vi "Goo01.vi"() -> ()   [LabVIEW 2014]
uses:
  <vilib>/myRIO/Instrument Drivers/Onboard IO/AI/vis/Read.vi
  <vilib>/myRIO/Instrument Drivers/Onboard IO/AI/vis/Smart Open.vi
  <vilib>/Utility/error.llb/Error Cluster From Error Code.vi
  <vilib>/myRIO/Common/Instrument Driver Framework/myRIO v1.0/AI/vis/myRIO v1.0 Read AI.vi
panel:
  out "웨이브폼 차트":cluster{"Col01 (B/AI1 (Pin 5))":dbl, dbl}(graph)
  out "숫자형":dbl=2.943114933
  out "Col02 (B/AI2 (Pin 7))":dbl=2.980956726
  out "원소의 인덱스":i32
  out "숫자형 2":dbl=2.46582006
  out "Col02 (B/AI2 (Pin 7)) 2":dbl=2.708739957
  # "오른쪽 수평 맞추기"
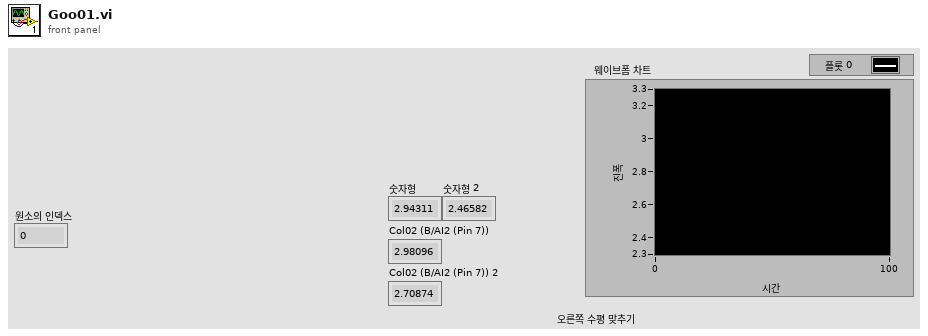
[diagram p1: front panel]
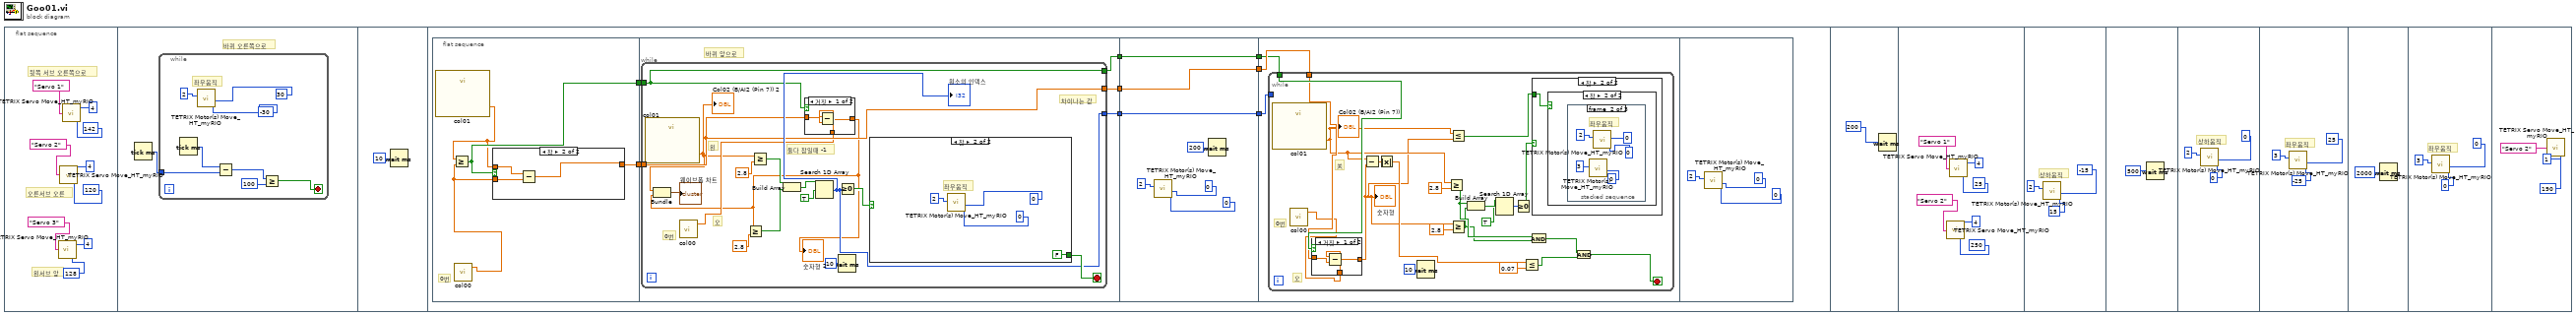
[diagram p0: block diagram]
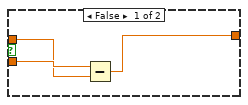
[diagram p2: hidden frame]
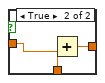
[diagram p3: hidden frame]
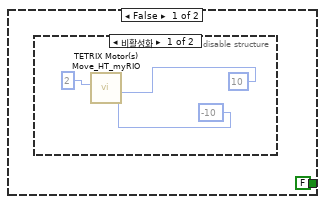
[diagram p4: hidden frame]
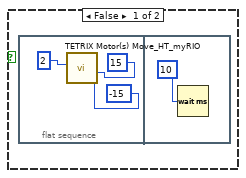
[diagram p6: hidden frame]
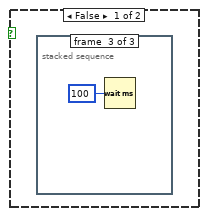
[diagram p7: hidden frame]
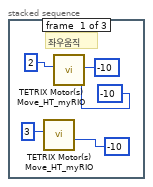
[diagram p8: hidden frame]
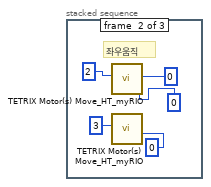
[diagram p9: hidden frame]
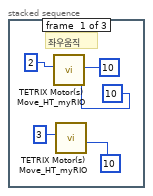
[diagram p10: hidden frame]
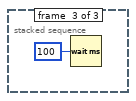
[diagram p11: hidden frame]
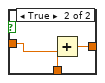
[diagram p12: hidden frame]
diagram:
  n1 = flat-sequence {
    frame #0 {
      # "왼서브 앞"
      # "오른서브 오른"
      # "뒷쪽 서브 오른쪽으로"
      n2 = call <vilib>:"TETRIX Servo Move_HT_myRIO.vi"("Servo Position (0 - 255)"=u8 128, "Controller Daisy Chain Position (1 - 4)"=u8 4, "Select Servo"="Servo 3") -> ()  [unwired: 2 in, 1 out]
      n3 = call <vilib>:"TETRIX Servo Move_HT_myRIO.vi"("Servo Position (0 - 255)"=u8 120, "Controller Daisy Chain Position (1 - 4)"=u8 4, "Select Servo"="Servo 2") -> ()  [unwired: 2 in, 1 out]
      n4 = call <vilib>:"TETRIX Servo Move_HT_myRIO.vi"("Servo Position (0 - 255)"=u8 142, "Controller Daisy Chain Position (1 - 4)"=u8 4, "Select Servo"="Servo 1") -> ()  [unwired: 2 in, 1 out]
    }
    frame #1 {
      # "바퀴 오른쪽으로"
      n5 = Tick Count (ms)() -> (millisecond timer value=w10:u32)
      n6 = while {
        tunnel: w10 -> [w14]
        stop <- w11 stop-if-true
        # "좌우움직"
        n7 = Tick Count (ms)() -> (millisecond timer value=w15:u32)
        n8 = call <vilib>:"TETRIX Motor(s) Move_HT_myRIO.vi"("Motor 2 Power (-100 to 100)\n0 = Stop/Brake\n-128 = Stop/Coast"=i8 -30 ("Motor 2 Power (-100 to 100)\n0 = Stop/Brake\n-128 = Stop/Coast"), "Motor 1 Power (-100 to 100)\n0 = Stop/Brake\n-128 = Stop/Coast"=i8 30 ("Motor 1 Power (-100 to 100)\n0 = Stop/Brake\n-128 = Stop/Coast"), "Controller Daisy Chain Position: 1 - 4"=u8 2) -> ()  [unwired: 6 in, 1 out]
        n9 = Subtract(x=w15, y=w14) -> (x-y=w13:u32)
        n10 = Greater Or Equal?(x=w13, y=u32 100) -> (x >= y?=w11:bool)
      }
    }
    frame #2 {
      n11 = Wait (ms)(milliseconds to wait=u32 10 ("대기 시간(ms)")) -> ()  [unwired: 1 out]
    }
    frame #3 {
      n12 = flat-sequence {
        tunnel: [w31] -> w27
        tunnel: [w30] -> w26
        tunnel: [w42] -> w25
        tunnel: [w41] -> w24
        tunnel: [w40] -> w23
        tunnel: w27 -> [w39]
        tunnel: w26 -> [w38]
        tunnel: w25 -> [w75]
        tunnel: w24 -> [w73]
        tunnel: w23 -> [w74]
        tunnel: [w75] -> w22
        tunnel: [w74] -> w21
        tunnel: [w73] -> w20
        tunnel: w22 -> [w82]
        tunnel: w21 -> [w81]
        tunnel: w20 -> [w80]
        frame #0 {
          # "0번"
          n13 = call "col01.vi"() -> ("Col01 (B/AI1 (Pin 5))"=w29:dbl)  [unwired: 26 in, 1 out]
          n14 = call "col00.vi"() -> ("Col00 (B/AI0 (Pin 3))"=w28:dbl)  [unwired: 26 in, 1 out]
          n15 = Greater Or Equal?(x=w29, y=w28) -> (x >= y?=w31:bool)
          n16 = case shown="참" w31 {
            tunnel: w29 -> [w33 w37]
            tunnel: w28 -> [w34 w36]
            tunnel: [w32 w35] -> w30
            frame False {
              n17 = Subtract(x=w34, y=w33) -> (x-y=w32:dbl)
            }
            frame True {
              n18 = Subtract(x=w37, y=w36) -> (x-y=w35:dbl)
            }
          }
        }
        frame #1 {
          # "바퀴 앞으로"
          n19 = while {
            tunnel: [w50] -> w42
            tunnel: [w48] -> w41
            tunnel: [w47] -> w40
            tunnel: w39 -> [w48]
            tunnel: w38 -> [w47]
            stop <- w51 stop-if-true
            # "0번"
            # "차이나는 값"
            # "오"
            # "왼"
            # "둘다 참일때 -1"
            n20 = call "col01.vi"() -> ("Col01 (B/AI1 (Pin 5))"=w43:dbl)  [unwired: 26 in, 1 out]
            "Col02 (B/AI2 (Pin 7)) 2" <- w43
            n21 = call "col00.vi"() -> ("Col00 (B/AI0 (Pin 3))"=w46:dbl)  [unwired: 26 in, 1 out]
            n22 = Greater Or Equal?(x=w43, y=2.8) -> (x >= y?=w54:bool)
            n23 = case shown="거짓" w48 {
              tunnel: w47 -> [w61 w64]
              tunnel: w46 -> [w60 w63]
              tunnel: [w59 w62] -> w44
              frame False {
                n24 = Subtract(x=w60, y=w61) -> (x-y=w59:dbl)
              }
              frame True {
                n25 = Add(x=w63, y=w64) -> (x+y=w62:dbl)
              }
            }
            "숫자형 2" <- w44
            n26 = Bundle("Col01 (B/AI1 (Pin 5))"=w43, w44) -> (→"웨이브폼 차트":cluster{"Col01 (B/AI1 (Pin 5))":dbl, dbl})  [unwired: 1 in]
            n27 = Greater Or Equal?(x=w44, y=2.8) -> (x >= y?=w55:bool)
            n28 = Build Array(w54, w55) -> (w58:bool[])
            n29 = Search 1D Array(1D array=w58, element=TRUE ("원소")) -> (index of element=w50:i32)  [unwired: 1 in]
            "원소의 인덱스" <- w50
            n30 = Wait (ms)(milliseconds to wait=u32 10 ("대기 시간(ms)")) -> ()  [unwired: 1 out]
            n31 = Greater Or Equal To 0?(x=w50) -> (x >= 0?=w56:bool)
            n32 = case shown="참" w56 {
              tunnel: [FALSE FALSE] -> w51
              frame False {
                n33 = disable-structure shown="비활성화" {
                  frame Disabled {
                    n34 = call <vilib>:"TETRIX Motor(s) Move_HT_myRIO.vi"("Motor 2 Power (-100 to 100)\n0 = Stop/Brake\n-128 = Stop/Coast"=i8 -10 ("Motor 2 Power (-100 to 100)\n0 = Stop/Brake\n-128 = Stop/Coast"), "Motor 1 Power (-100 to 100)\n0 = Stop/Brake\n-128 = Stop/Coast"=i8 10 ("Motor 1 Power (-100 to 100)\n0 = Stop/Brake\n-128 = Stop/Coast"), "Controller Daisy Chain Position: 1 - 4"=u8 2) -> ()  [unwired: 6 in, 1 out]
                  }
                  frame Enabled {
                  }
                }
              }
              frame True {
                # "좌우움직"
                n35 = call <vilib>:"TETRIX Motor(s) Move_HT_myRIO.vi"("Motor 2 Power (-100 to 100)\n0 = Stop/Brake\n-128 = Stop/Coast"=i8 0 ("Motor 2 Power (-100 to 100)\n0 = Stop/Brake\n-128 = Stop/Coast"), "Motor 1 Power (-100 to 100)\n0 = Stop/Brake\n-128 = Stop/Coast"=i8 0 ("Motor 1 Power (-100 to 100)\n0 = Stop/Brake\n-128 = Stop/Coast"), "Controller Daisy Chain Position: 1 - 4"=u8 2) -> ()  [unwired: 6 in, 1 out]
              }
            }
          }
        }
        frame #2 {
          n36 = call <vilib>:"TETRIX Motor(s) Move_HT_myRIO.vi"("Motor 2 Power (-100 to 100)\n0 = Stop/Brake\n-128 = Stop/Coast"=i8 0 ("Motor 2 Power (-100 to 100)\n0 = Stop/Brake\n-128 = Stop/Coast"), "Motor 1 Power (-100 to 100)\n0 = Stop/Brake\n-128 = Stop/Coast"=i8 0 ("Motor 1 Power (-100 to 100)\n0 = Stop/Brake\n-128 = Stop/Coast"), "Controller Daisy Chain Position: 1 - 4"=u8 2) -> ()  [unwired: 6 in, 1 out]
          n37 = Wait (ms)(milliseconds to wait=u32 200 ("대기 시간(ms)")) -> ()  [unwired: 1 out]
        }
        frame #3 {
          n38 = while {
            tunnel: w82 -> [_]
            tunnel: w80 -> [w102]
            tunnel: w81 -> [w101]
            stop <- w95 stop-if-true
            # "0번"
            # "오"
            # "关"
            n39 = call "col01.vi"() -> ("Col01 (B/AI1 (Pin 5))"=w85:dbl)  [unwired: 26 in, 1 out]
            "Col02 (B/AI2 (Pin 7))" <- w85
            n40 = call "col00.vi"() -> ("Col00 (B/AI0 (Pin 3))"=w93:dbl)  [unwired: 26 in, 1 out]
            n41 = case shown="거짓" w102 {
              tunnel: w101 -> [w133 w136]
              tunnel: w93 -> [w132 w135]
              tunnel: [w131 w134] -> w84
              frame False {
                n42 = Subtract(x=w132, y=w133) -> (x-y=w131:dbl)
              }
              frame True {
                n43 = Add(x=w135, y=w136) -> (x+y=w134:dbl)
              }
            }
            "숫자형" <- w84
            n44 = Subtract(x=w85, y=w84) -> (x-y=w103:dbl)
            n45 = Absolute Value(x=w103) -> (abs(x)=w90:dbl)
            n46 = Wait (ms)(milliseconds to wait=u32 10 ("대기 시간(ms)")) -> ()  [unwired: 1 out]
            n47 = Greater Or Equal?(x=w85, y=2.8) -> (x >= y?=w88:bool)
            n48 = Less Or Equal?(x=w85, y=w84) -> (x <= y?=w83:bool)
            n49 = Greater Or Equal?(x=w84, y=2.8) -> (x >= y?=w87:bool)
            n50 = Build Array(w88, w87) -> (w97:bool[])
            n51 = Search 1D Array(1D array=w97, element=TRUE ("원소")) -> (index of element=w94:i32)  [unwired: 1 in]
            n52 = Greater Or Equal To 0?(x=w94) -> (x >= 0?=w92:bool)
            n53 = Less Or Equal?(x=w90, y=0.07) -> (x <= y?=w91:bool)
            n54 = And(x=w88, y=w87) -> (x .and. y?=w86:bool)
            n55 = case shown="참" w92 {
              tunnel: w83 -> [_ w108]
              frame False {
                n56 = flat-sequence {
                  frame #0 {
                    n57 = call <vilib>:"TETRIX Motor(s) Move_HT_myRIO.vi"("Motor 2 Power (-100 to 100)\n0 = Stop/Brake\n-128 = Stop/Coast"=i8 -15 ("Motor 2 Power (-100 to 100)\n0 = Stop/Brake\n-128 = Stop/Coast"), "Motor 1 Power (-100 to 100)\n0 = Stop/Brake\n-128 = Stop/Coast"=i8 15 ("Motor 1 Power (-100 to 100)\n0 = Stop/Brake\n-128 = Stop/Coast"), "Controller Daisy Chain Position: 1 - 4"=u8 2) -> ()  [unwired: 6 in, 1 out]
                  }
                  frame #1 {
                    n58 = Wait (ms)(milliseconds to wait=u32 10 ("ms 타이머 값")) -> ()  [unwired: 1 out]
                  }
                }
              }
              frame True {
                n59 = case shown="참" w108 {
                  frame False {
                    n60 = stacked-sequence {
                      frame #0 {
                        # "좌우움직"
                        n61 = call <vilib>:"TETRIX Motor(s) Move_HT_myRIO.vi"("Motor 1 Power (-100 to 100)\n0 = Stop/Brake\n-128 = Stop/Coast"=i8 -10 ("Motor 1 Power (-100 to 100)\n0 = Stop/Brake\n-128 = Stop/Coast"), "Controller Daisy Chain Position: 1 - 4"=u8 3) -> ()  [unwired: 7 in, 1 out]
                        n62 = call <vilib>:"TETRIX Motor(s) Move_HT_myRIO.vi"("Motor 2 Power (-100 to 100)\n0 = Stop/Brake\n-128 = Stop/Coast"=i8 -10 ("Motor 2 Power (-100 to 100)\n0 = Stop/Brake\n-128 = Stop/Coast"), "Motor 1 Power (-100 to 100)\n0 = Stop/Brake\n-128 = Stop/Coast"=i8 -10 ("Motor 1 Power (-100 to 100)\n0 = Stop/Brake\n-128 = Stop/Coast"), "Controller Daisy Chain Position: 1 - 4"=u8 2) -> ()  [unwired: 6 in, 1 out]
                      }
                      frame #1 {
                        # "좌우움직"
                        n63 = call <vilib>:"TETRIX Motor(s) Move_HT_myRIO.vi"("Motor 2 Power (-100 to 100)\n0 = Stop/Brake\n-128 = Stop/Coast"=i8 0 ("Motor 2 Power (-100 to 100)\n0 = Stop/Brake\n-128 = Stop/Coast"), "Motor 1 Power (-100 to 100)\n0 = Stop/Brake\n-128 = Stop/Coast"=i8 0 ("Motor 1 Power (-100 to 100)\n0 = Stop/Brake\n-128 = Stop/Coast"), "Controller Daisy Chain Position: 1 - 4"=u8 2) -> ()  [unwired: 6 in, 1 out]
                        n64 = call <vilib>:"TETRIX Motor(s) Move_HT_myRIO.vi"("Motor 1 Power (-100 to 100)\n0 = Stop/Brake\n-128 = Stop/Coast"=i8 0 ("Motor 1 Power (-100 to 100)\n0 = Stop/Brake\n-128 = Stop/Coast"), "Controller Daisy Chain Position: 1 - 4"=u8 3) -> ()  [unwired: 7 in, 1 out]
                      }
                      frame #2 {
                        n65 = Wait (ms)(milliseconds to wait=u32 100 ("대기 시간(ms)")) -> ()  [unwired: 1 out]
                      }
                    }
                  }
                  frame True {
                    n66 = stacked-sequence {
                      frame #0 {
                        # "좌우움직"
                        n67 = call <vilib>:"TETRIX Motor(s) Move_HT_myRIO.vi"("Motor 2 Power (-100 to 100)\n0 = Stop/Brake\n-128 = Stop/Coast"=i8 10 ("Motor 2 Power (-100 to 100)\n0 = Stop/Brake\n-128 = Stop/Coast"), "Motor 1 Power (-100 to 100)\n0 = Stop/Brake\n-128 = Stop/Coast"=i8 10 ("Motor 1 Power (-100 to 100)\n0 = Stop/Brake\n-128 = Stop/Coast"), "Controller Daisy Chain Position: 1 - 4"=u8 2) -> ()  [unwired: 6 in, 1 out]
                        n68 = call <vilib>:"TETRIX Motor(s) Move_HT_myRIO.vi"("Motor 1 Power (-100 to 100)\n0 = Stop/Brake\n-128 = Stop/Coast"=i8 10 ("Motor 1 Power (-100 to 100)\n0 = Stop/Brake\n-128 = Stop/Coast"), "Controller Daisy Chain Position: 1 - 4"=u8 3) -> ()  [unwired: 7 in, 1 out]
                      }
                      frame #1 {
                        # "좌우움직"
                        n69 = call <vilib>:"TETRIX Motor(s) Move_HT_myRIO.vi"("Motor 1 Power (-100 to 100)\n0 = Stop/Brake\n-128 = Stop/Coast"=i8 0 ("Motor 1 Power (-100 to 100)\n0 = Stop/Brake\n-128 = Stop/Coast"), "Controller Daisy Chain Position: 1 - 4"=u8 3) -> ()  [unwired: 7 in, 1 out]
                        n70 = call <vilib>:"TETRIX Motor(s) Move_HT_myRIO.vi"("Motor 2 Power (-100 to 100)\n0 = Stop/Brake\n-128 = Stop/Coast"=i8 0 ("Motor 2 Power (-100 to 100)\n0 = Stop/Brake\n-128 = Stop/Coast"), "Motor 1 Power (-100 to 100)\n0 = Stop/Brake\n-128 = Stop/Coast"=i8 0 ("Motor 1 Power (-100 to 100)\n0 = Stop/Brake\n-128 = Stop/Coast"), "Controller Daisy Chain Position: 1 - 4"=u8 2) -> ()  [unwired: 6 in, 1 out]
                      }
                      frame #2 {
                        n71 = Wait (ms)(milliseconds to wait=u32 100 ("대기 시간(ms)")) -> ()  [unwired: 1 out]
                      }
                    }
                  }
                }
              }
            }
            n72 = And(x=w86, y=w91) -> (x .and. y?=w95:bool)
          }
        }
        frame #4 {
          n73 = call <vilib>:"TETRIX Motor(s) Move_HT_myRIO.vi"("Motor 2 Power (-100 to 100)\n0 = Stop/Brake\n-128 = Stop/Coast"=i8 0 ("Motor 2 Power (-100 to 100)\n0 = Stop/Brake\n-128 = Stop/Coast"), "Motor 1 Power (-100 to 100)\n0 = Stop/Brake\n-128 = Stop/Coast"=i8 0 ("Motor 1 Power (-100 to 100)\n0 = Stop/Brake\n-128 = Stop/Coast"), "Controller Daisy Chain Position: 1 - 4"=u8 2) -> ()  [unwired: 6 in, 1 out]
        }
      }
    }
    frame #4 {
      n74 = Wait (ms)(milliseconds to wait=u32 200 ("대기 시간(ms)")) -> ()  [unwired: 1 out]
    }
    frame #5 {
      n75 = call <vilib>:"TETRIX Servo Move_HT_myRIO.vi"("Servo Position (0 - 255)"=u8 250, "Controller Daisy Chain Position (1 - 4)"=u8 4, "Select Servo"="Servo 2") -> ()  [unwired: 2 in, 1 out]
      n76 = call <vilib>:"TETRIX Servo Move_HT_myRIO.vi"("Servo Position (0 - 255)"=u8 25, "Controller Daisy Chain Position (1 - 4)"=u8 4, "Select Servo"="Servo 1") -> ()  [unwired: 2 in, 1 out]
    }
    frame #6 {
      # "상하움직"
      n77 = call <vilib>:"TETRIX Motor(s) Move_HT_myRIO.vi"("Motor 2 Power (-100 to 100)\n0 = Stop/Brake\n-128 = Stop/Coast"=i8 15 ("Motor 2 Power (-100 to 100)\n0 = Stop/Brake\n-128 = Stop/Coast"), "Motor 1 Power (-100 to 100)\n0 = Stop/Brake\n-128 = Stop/Coast"=i8 -15 ("Motor 1 Power (-100 to 100)\n0 = Stop/Brake\n-128 = Stop/Coast"), "Controller Daisy Chain Position: 1 - 4"=u8 2) -> ()  [unwired: 6 in, 1 out]
    }
    frame #7 {
      n78 = Wait (ms)(milliseconds to wait=u32 500 ("대기 시간(ms)")) -> ()  [unwired: 1 out]
    }
    frame #8 {
      # "상하움직"
      n79 = call <vilib>:"TETRIX Motor(s) Move_HT_myRIO.vi"("Motor 2 Power (-100 to 100)\n0 = Stop/Brake\n-128 = Stop/Coast"=i8 0 ("Motor 2 Power (-100 to 100)\n0 = Stop/Brake\n-128 = Stop/Coast"), "Motor 1 Power (-100 to 100)\n0 = Stop/Brake\n-128 = Stop/Coast"=i8 0 ("Motor 1 Power (-100 to 100)\n0 = Stop/Brake\n-128 = Stop/Coast"), "Controller Daisy Chain Position: 1 - 4"=u8 2) -> ()  [unwired: 6 in, 1 out]
    }
    frame #9 {
      # "좌우움직"
      n80 = call <vilib>:"TETRIX Motor(s) Move_HT_myRIO.vi"("Motor 2 Power (-100 to 100)\n0 = Stop/Brake\n-128 = Stop/Coast"=i8 -25 ("Motor 2 Power (-100 to 100)\n0 = Stop/Brake\n-128 = Stop/Coast"), "Motor 1 Power (-100 to 100)\n0 = Stop/Brake\n-128 = Stop/Coast"=i8 25 ("Motor 1 Power (-100 to 100)\n0 = Stop/Brake\n-128 = Stop/Coast"), "Controller Daisy Chain Position: 1 - 4"=u8 3) -> ()  [unwired: 6 in, 1 out]
    }
    frame #10 {
      n81 = Wait (ms)(milliseconds to wait=u32 2000 ("대기 시간(ms)")) -> ()  [unwired: 1 out]
    }
    frame #11 {
      # "좌우움직"
      n82 = call <vilib>:"TETRIX Motor(s) Move_HT_myRIO.vi"("Motor 2 Power (-100 to 100)\n0 = Stop/Brake\n-128 = Stop/Coast"=i8 0 ("Motor 2 Power (-100 to 100)\n0 = Stop/Brake\n-128 = Stop/Coast"), "Motor 1 Power (-100 to 100)\n0 = Stop/Brake\n-128 = Stop/Coast"=i8 0 ("Motor 1 Power (-100 to 100)\n0 = Stop/Brake\n-128 = Stop/Coast"), "Controller Daisy Chain Position: 1 - 4"=u8 3) -> ()  [unwired: 6 in, 1 out]
    }
    frame #12 {
      n83 = call <vilib>:"TETRIX Servo Move_HT_myRIO.vi"("Servo Position (0 - 255)"=u8 190, "Controller Daisy Chain Position (1 - 4)"=u8 1, "Select Servo"="Servo 2") -> ()  [unwired: 2 in, 1 out]
    }
  }
